vi "SubVI Tester.vi"() -> ()   [LabVIEW 2015]
uses:
  C:/Users/Student/Desktop/249556/Kody/Laboratorium 3/Weather Warnings/Weather Data.ctl
panel:
  out "Wheater data out":T1={"Current Temperature"=0.0, "Max Temperature"=0.0, "Min Temperature"=0.0, "Warning?"=FALSE, "Warning Text"="No Warning", "Units"=enum."Celsius"}
  in  "Min Temperature":dbl=10.0
  in  "Max Temperature":dbl=30.0
  in  "Stop":bool
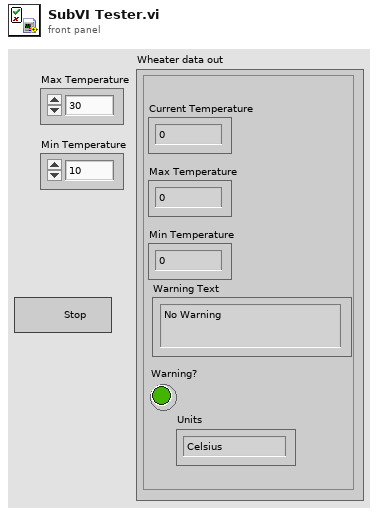
[diagram p1: front panel]
types:
  T1 = typedef "Weather Data.ctl" = cluster{"Current Temperature":dbl, "Max Temperature":dbl, "Min Temperature":dbl, "Warning?":bool, "Warning Text":string, "Units":enum16{"Celsius", "Fahrenheit"}}
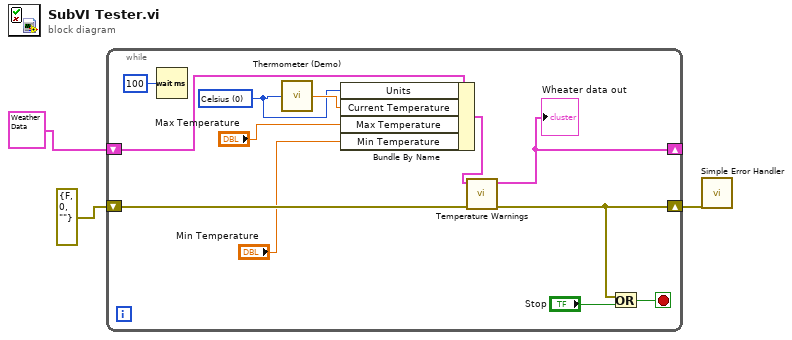
[diagram p0: block diagram]
diagram:
  n1 = while {
    shift-right: [w11] -> w3
    shift-left: errorcluster {"status"=FALSE, "code"=0, "source"=""} ("error out") -> [w12]
    shift-right: [w5] -> _
    shift-left: T1 {"Current Temperature"=0.0, "Max Temperature"=0.0, "Min Temperature"=0.0, "Warning?"=FALSE, "Warning Text"="No Warning", "Units"=enum."Celsius"} ("Wheater data in") -> [w7]
    stop <- w13 stop-if-true
    w4 = u16 0 items=["Celsius", "Fahrenheit"] ("Units (0: Celsius)")
    n2 = Wait (ms)(milliseconds to wait=u32 100) -> ()  [unwired: 1 out]
    n3 = call "Thermometer (Demo).vi"("Units (0: Celsius)"=w4) -> ("Temperature Value"=w10:dbl)
    n4 = Bundle By Name(cluster=w7, "Units"=w4, "Current Temperature"=w10, "Max Temperature"="Max Temperature", "Min Temperature"="Min Temperature") -> (w6:T1)
    n5 = call "Temperature Warnings.vi"("Error In"=w12, "Wheater data in"=w6) -> ("Error Out"=w11:errorcluster, "Wheater data out"=w5:T1)  [unwired: 8 in]
    "Wheater data out" <- w5
    n6 = Or(x=w11, y="Stop") -> (x .or. y?=w13:bool)
  }
  n7 = call <vilib>:"Simple Error Handler.vi"("error in (no error)"=w3) -> ()  [unwired: 4 in, 5 out]
